vi "Generate Log File.vi"(0 "Log Data":dbl[][](array[numeric]) format="%0.2f", 1 "Time":timestamp, 2 "Dropbox Directory":string) -> ()   [LabVIEW 2011]
uses:
  <vilib>/Utility/file.llb/Write To Spreadsheet File (DBL).vi
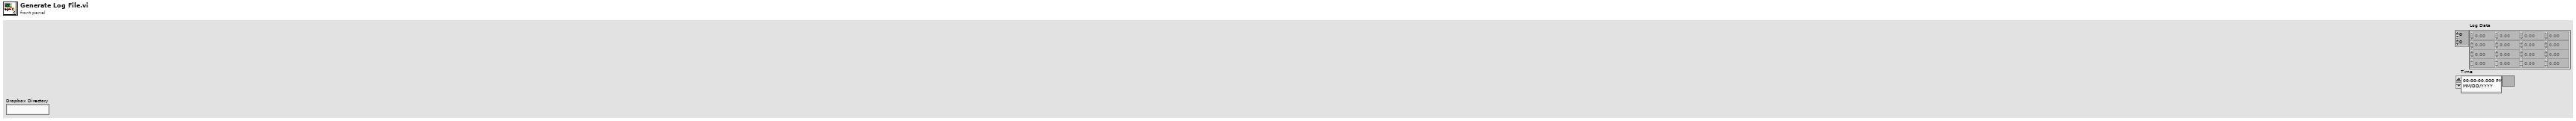
[diagram p1: front panel]
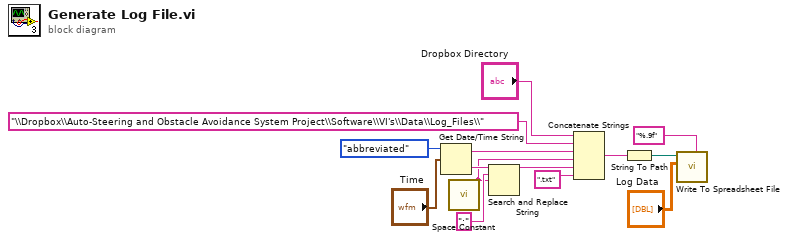
[diagram p0: block diagram]
diagram:
  n1 = Get Date/Time String(date format (0)=enum16{"short", "long", "abbreviated"}."abbreviated", seconds (now)="Time") -> (date string=w14:string, time string=w10:string)  [unwired: 1 in]
  n2 = call <vilib>:"Space Constant.vi"() -> ("String"=w8:string)
  n3 = Search and Replace String(input string=w10, search string=":", replace string=w8) -> (result string=w7:string)  [unwired: 5 in, 3 out]
  n4 = Concatenate Strings("Dropbox Directory", "\\Dropbox\\Auto-Steering and Obstacle Avoidance System Project\\Software\\VI's\\Data\\Log_Files\\" ("string"), w14, w8, w7, ".txt" ("string")) -> (w5:string)
  n5 = String To Path(string=w5) -> (path=w6:path)
  n6 = call-poly <vilib>:"Write To Spreadsheet File.vi"("format (%.3f)"="%.9f", "2D data"="Log Data", "file path (dialog if empty)"=w6) -> ()  [unwired: 5 in, 1 out]
